vi "Magnet_ID.vi"() -> (0 "Cell":string)   [LabVIEW 2020]
doc: "This searches the magnet calibrations folder and returns the ids of every magnet calibration file found.\nScott Hannahs, NHMFL - FSU, April 1998"
panel:
  out "Status":cluster{bool, bool, "Ramp Status":u16, bool}
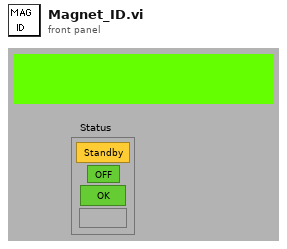
[diagram p1: front panel]
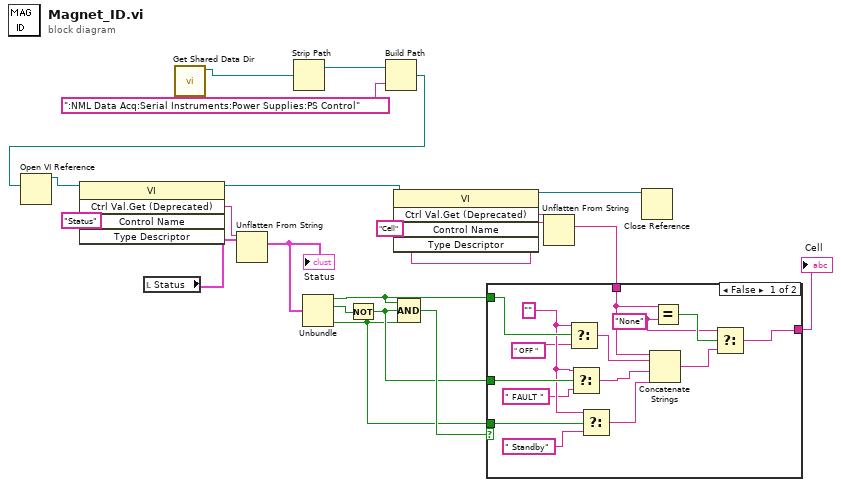
[diagram p0: block diagram]
diagram:
  w20 = "Cell" ("Control Name")
  n1 = local read "Status"() -> (w12:cluster{bool, bool, "Ramp Status":u16, bool})
  n2 = call "Get Shared Data Dir.vi"() -> ("Data Directory Path"=w2:path)  [unwired: 2 in, 1 out]
  n3 = Strip Path(path=w2) -> (stripped path=w1:path)  [unwired: 1 out]
  n4 = Build Path(base path=w1, name or relative path=":NML Data Acq:Serial Instruments:Power Supplies:PS Control") -> (appended path=w3:path)
  n5 = Open VI Reference(vi path=w3) -> (vi reference=w16:refnum<vi>)  [unwired: 5 in, 1 out]
  n6 = invoke class="VI" method="Ctrl Val.Get (Deprecated)"(reference=w16, "Control Name"="Status") -> (reference out=w15:refnum<vi>, "Get Control Value"=w13:string)  [unwired: 3 in, 3 out]
  n7 = Unflatten From String(type=w12, binary string=w13) -> (value=w11:cluster{bool, bool, "Ramp Status":u16, bool})  [unwired: 3 in, 2 out]
  "Status" <- w11
  n8 = Unbundle(w11) -> (w7:bool, w18:bool, w5:bool)  [unwired: 1 out]
  n9 = Not(x=w18) -> (.not. x?=w6:bool)
  n10 = invoke class="VI" method="Ctrl Val.Get (Deprecated)"(reference=w15, "Control Name"=w20) -> (reference out=w17:refnum<vi>, "Get Control Value"=w19:string)  [unwired: 3 in, 3 out]
  n11 = Compound Arithmetic op=AND(w7, w6, w5) -> (w10:bool)
  n12 = Unflatten From String(type=w20, binary string=w19) -> (value=w8:string)  [unwired: 3 in, 2 out]
  n13 = case shown="False" w10 {
    tunnel: [w21 w36] -> w9
    tunnel: w8 -> [w23 w36]
    tunnel: w7 -> [w35 _]
    tunnel: w6 -> [w34 _]
    tunnel: w5 -> [w33 _]
    frame False {
      w32 = "" ("Cell")
      w24 = "None" ("Cell")
      n14 = Select(t=w32, s=w35, f=" OFF " ("Cell")) -> (s? t:f=w28:string)
      n15 = Select(t=w32, s=w34, f=" FAULT " ("Cell")) -> (s? t:f=w27:string)
      n16 = Select(t=w32, s=w33, f=" Standby" ("Cell")) -> (s? t:f=w26:string)
      n17 = Concatenate Strings(w23, w28, w27, w26) -> (w22:string)
      n18 = Equal?(x=w23, y=w24) -> (x = y?=w25:bool)
      n19 = Select(t=w24, s=w25, f=w22) -> (s? t:f=w21:string)
    }
    frame True {
    }
  }
  "Cell" <- w9
  n20 = Close Reference(reference=w17) -> ()  [unwired: 1 in, 1 out]
